vi "VarParFormats.vi"(8 "ErrorIn(No Error)":errorcluster caption="entrée d'erreur (pas d'erreur)", 9 "IndCourbe":i64, 10 "InstrumentName":string, 11 "VarParArr":string[][](array[string])) -> (0 "Err Out":errorcluster caption="sortie d'erreur", 3 "VarParArrOut":string[][](array[string]))   [LabVIEW 2019]
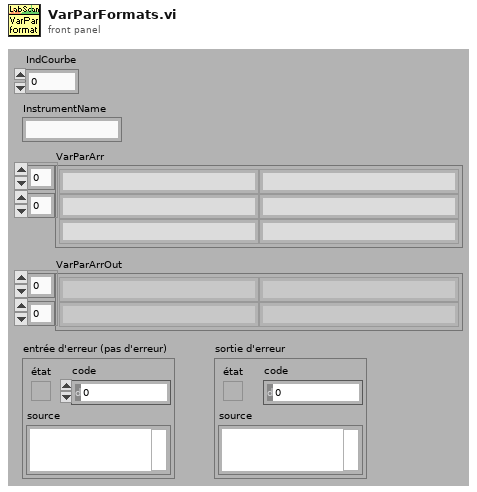
[diagram p1: front panel]
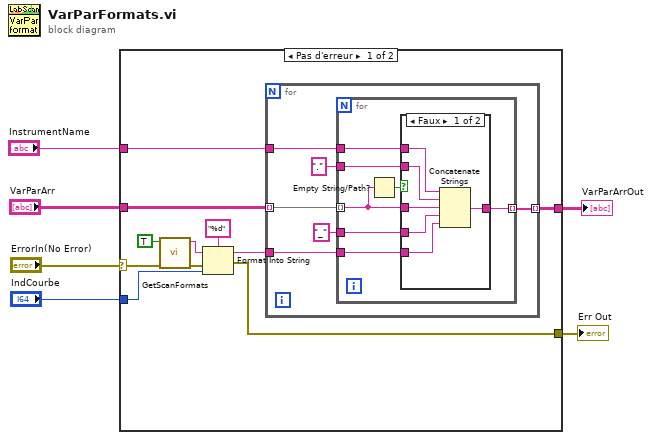
[diagram p0: block diagram]
diagram:
  n1 = case shown="Pas d'erreur" "ErrorIn(No Error)" {
    selector: "ErrorIn(No Error)" -> [w10 w38]
    tunnel: [w8 w38] -> w5
    tunnel: "IndCourbe" -> [w13 _]
    tunnel: "InstrumentName" -> [w12 _]
    tunnel: "VarParArr" -> [w11 _]
    tunnel: [w7 _] -> w1
    frame No Error {
      n2 = call "GetScanFormats.vi"("ErrorIn(No Error)"=w10, "Scan(T)"=TRUE) -> ("sortie d'erreur"=w9:errorcluster, "Prefixe"=w15:string)  [unwired: 7 in, 1 out]
      n3 = Format Into String(format string="%d" ("chaîne de format"), initial string=w15, error in=w9, w13) -> (resulting string=w14:string, error out=w8:errorcluster)
      n4 = for {
        tunnel: [w23] -> w7 mode=indexing
        tunnel: w12 -> [w22]
        tunnel: w11 -> [w21] mode=indexing
        tunnel: w14 -> [w20]
        n5 = for {
          tunnel: w21 -> [w24] mode=indexing
          tunnel: "." ("chaîne") -> [w30]
          tunnel: [w29] -> w23 mode=indexing
          tunnel: w22 -> [w28]
          tunnel: "_" ("chaîne") -> [w26]
          tunnel: w20 -> [w27]
          n6 = Empty String/Path?(string/path=w24) -> (empty?=w25:bool)
          n7 = case shown="Faux" w25 {
            tunnel: w24 -> [w36 w37]
            tunnel: w30 -> [w35 _]
            tunnel: [w34 w37] -> w29
            tunnel: w28 -> [w33 _]
            tunnel: w27 -> [w32 _]
            tunnel: w26 -> [w31 _]
            frame False {
              n8 = Concatenate Strings(w33, w35, w36, w31, w32) -> (w34:string)
            }
            frame True {
            }
          }
        }
      }
    }
    frame Error {
    }
  }
  "Err Out" <- w5
  "VarParArrOut" <- w1
